vi "Read VI Ref.vi"(8 "error in (no error)":errorcluster, 11 "Chart in":refnum<class "Chart.lvclass">) -> (0 "error out":errorcluster, 2 "VI Ref":refnum<vi>, 3 "Chart out":refnum<class "Chart.lvclass">)   [LabVIEW 2021, in "Chart.lvclass"]
doc: "This VI reads Chart VI Ref."
uses:
  Chart.lvclass
  Chart.lvclass/Chart.ctl
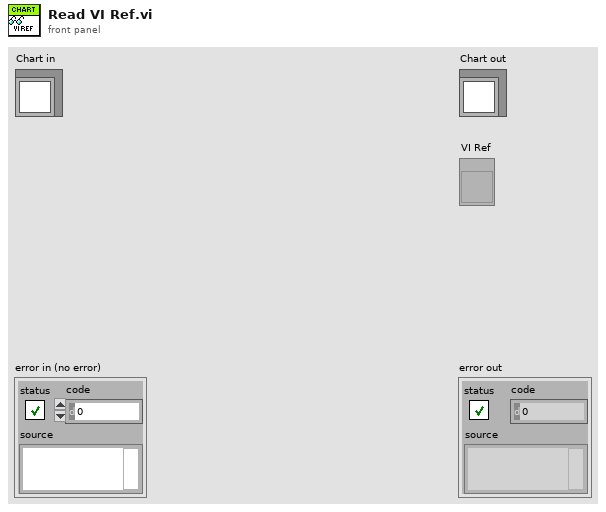
[diagram p1: front panel]
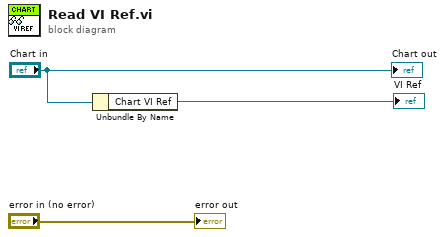
[diagram p0: block diagram]
diagram:
  n1 = Unbundle By Name("Chart in") -> ("Chart VI Ref"=→"VI Ref":refnum<vi>)
  "error out" <- "error in (no error)"
  "Chart out" <- "Chart in"
